vi "启动参数设置.vi"() -> ()   [LabVIEW 2016, in "斯坦道氨氮.lvlib"]
uses:
  <vilib>/Utility/miscctls.llb/LVPointTypeDef.ctl
  <vilib>/Utility/config.llb/NI_LVConfig.lvlib
panel:
  in  "启动参数":T1
  in  "取消":bool
  in  "确认":bool
  # "请选择启动参数"
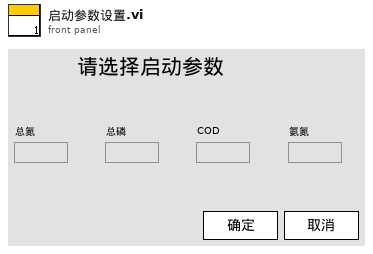
[diagram p1: front panel]
types:
  T1 = cluster{"COD":bool, "氨氮":bool, "总氮":bool, "总磷":bool}
  T2 = typedef "LVPointTypeDef.ctl" = cluster{"Horizontal":i16, "Vertical":i16}
  T3 = typedef "NI_LVConfig.lvlib/Config Data RefNum.ctl" = refnum<k1>
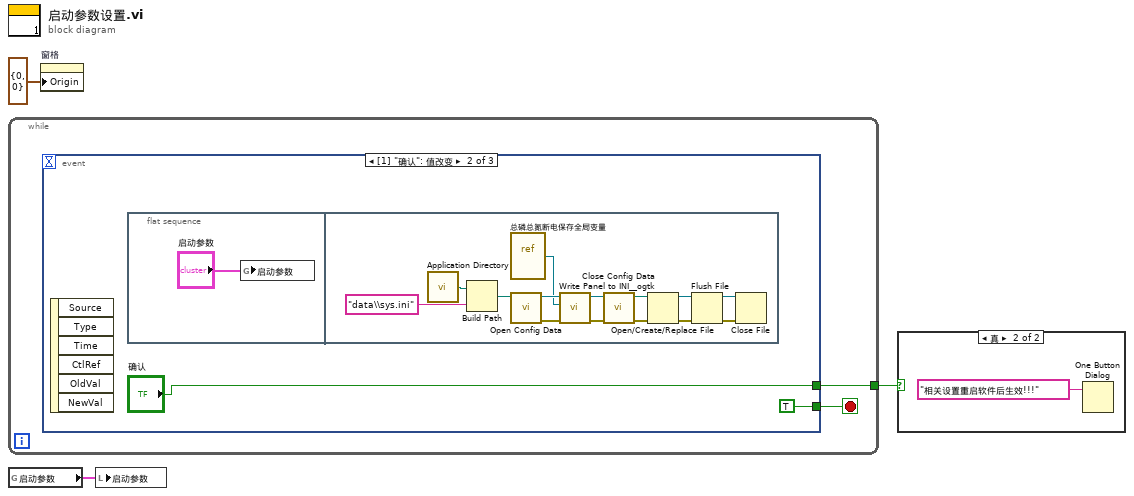
[diagram p0: block diagram]
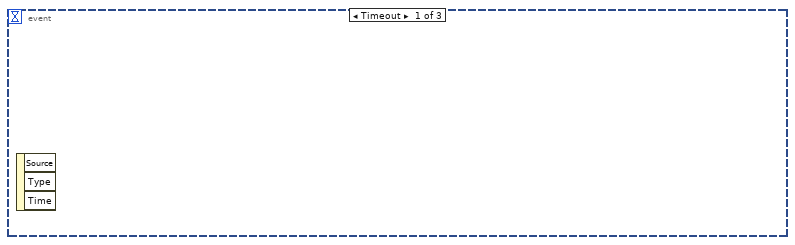
[diagram p3: hidden frame]
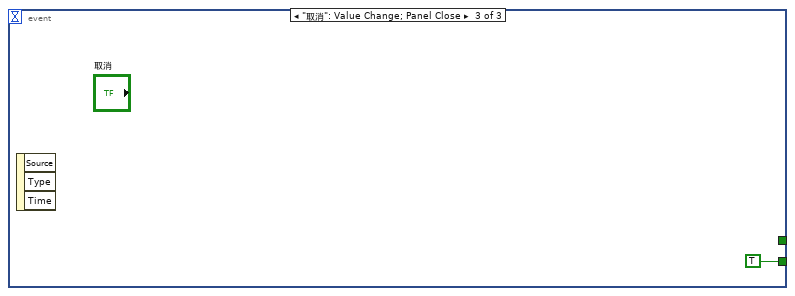
[diagram p4: hidden frame]
diagram:
  n1 = while {
    tunnel: [w4] -> w1
    stop <- w5 stop-if-true
    n2 = event shown="[1] \"确认\": 值改变" {
      selector: _ -> [_ _ _]
      dyn-events: _ -> [_ _ _]
      timeout: _ -> [_ _ _]
      tunnel: [_ TRUE TRUE] -> w5
      tunnel: [_ "确认" _] -> w4
      event Timeout {
        n3 = event-data() -> ()  [unwired: 1 in, 3 out]
      }
      event "确认": Value Change {
        n4 = event-data() -> ()  [unwired: 1 in, 6 out]
        n5 = flat-sequence {
          frame #0 {
            n6 = global write "总磷总氮断电保存全局变量.vi" "启动参数"("启动参数") -> ()
          }
          frame #1 {
            n7 = call <vilib>:"Application Directory.vi"() -> ("Application Directory"=w22:path)
            n8 = Build Path(base path=w22, name or relative path="data\\sys.ini" ("名称或相对路径")) -> (appended path=w20:path)
            n9 = vi-ref "总磷总氮断电保存全局变量.vi"() -> (w18:refnum<vi>)
            n10 = call <vilib>:"Open Config Data.vi"("configuration file path"=w20) -> ("error out"=w16:errorcluster, "refnum"=w19:T3)  [unwired: 8 in, 1 out]
            n11 = call <userlib>:"Write Panel to INI__ogtk.vi"("error in (no error)"=w16, "VI ref"=w18, "refnum"=w19) -> ("error out"=w15:errorcluster, "refnum out"=w17:T3)  [unwired: 7 in]
            n12 = call <vilib>:"Close Config Data.vi"("error in (no error)"=w15, "refnum"=w17) -> ("error out"=w10:errorcluster, "file path"=w9:path)  [unwired: 8 in]
            n13 = Open/Create/Replace File(file path (use dialog)=w9, error in=w10) -> (refnum out=w13:refnum<file>, error out=w14:errorcluster)  [unwired: 4 in, 1 out]
            n14 = Flush File(refnum=w13, error in=w14) -> (refnum out=w12:refnum<file>, error out=w11:errorcluster)
            n15 = Close File(refnum=w12, error in=w11) -> ()  [unwired: 2 out]
          }
        }
      }
      event "取消": Value Change; Panel Close {
        n16 = event-data() -> ()  [unwired: 1 in, 3 out]
      }
    }
  }
  n17 = global read "总磷总氮断电保存全局变量.vi" "启动参数"() -> (w2:T1)
  n18 = property on="窗格" class="Pane"("Origin"=T2 {"Horizontal"=0, "Vertical"=0} ("原点")) -> ()  [unwired: 2 in, 2 out]
  n19 = local write "启动参数"(w2) -> ()
  n20 = case shown="真" w1 {
    frame False {
    }
    frame True {
      n21 = One Button Dialog(message="相关设置重启软件后生效!!!" ("按钮名称（“确定”）")) -> ()  [unwired: 1 in, 1 out]
    }
  }
